vi "Set Position.vi"(8 "error in (no error)":errorcluster, 9 "Datum":T1, 10 "Target Coordinates":T2, 11 "Flex UI (Actor) in":refnum<class "Flex UI (Actor).lvclass">) -> (0 "error out":errorcluster, 3 "Flex UI (Actor) out":refnum<class "Flex UI (Actor).lvclass">)   [LabVIEW 2016, in "Flex UI (Parent Actor).lvlib" / "Flex UI (Actor).lvclass"]
doc: "Wrapper around the set position Flex UI class method."
uses:
  Flex UI (Actor).lvclass
  <vilib>/Utility/miscctls.llb/LVPositionTypeDef.ctl
  <vilib>/East West Architects/Flex UI/Flex UI (Parent)/Enum - Datum.ctl
  <vilib>/East West Architects/Flex UI/Flex UI (Parent)/Flex UI.lvclass
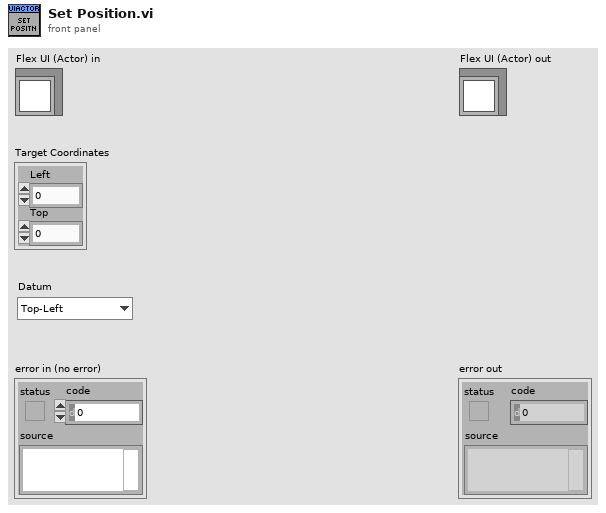
[diagram p1: front panel]
types:
  T1 = typedef "Flex UI.lvclass/Enum - Datum.ctl" = enum16{"Top-Left", "Top-Right", "Bottom-Left", "Bottom-Right", "Center"}
  T2 = typedef "LVPositionTypeDef.ctl" = cluster{"Left":i32, "Top":i32}
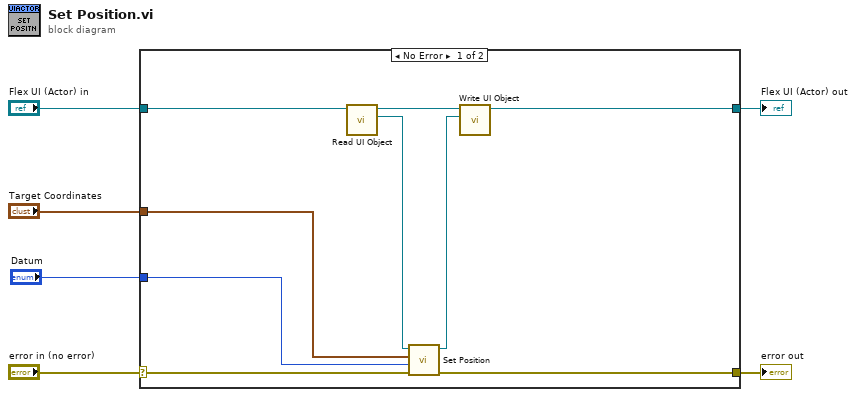
[diagram p0: block diagram]
diagram:
  n1 = case shown="No Error" "error in (no error)" {
    selector: "error in (no error)" -> [w14 w17]
    tunnel: [w13 w17] -> w5
    tunnel: [w10 w16] -> w3
    tunnel: "Flex UI (Actor) in" -> [w15 w16]
    tunnel: "Target Coordinates" -> [w8 _]
    tunnel: "Datum" -> [w7 _]
    frame No Error {
      n2 = call-dynamic "Read UI Object.vi"("Flex UI (Actor) in"=w15) -> ("Flex UI Object"=w11:refnum<class "Flex UI.lvclass">, "Flex UI (Actor) out"=w12:refnum<class "Flex UI (Actor).lvclass">)  [unwired: 8 in, 1 out]
      n3 = call-dynamic "Set Position.vi"("error in"=w14, "Datum"=w7, "Target Coordinates"=w8, "Flex UI in"=w11) -> ("error out"=w13:errorcluster, "Flex UI out"=w9:refnum<class "Flex UI.lvclass">)  [unwired: 6 in]
      n4 = call-dynamic "Write UI Object.vi"("Flex UI in"=w9, "Flex UI (Actor) in"=w12) -> ("Flex UI (Actor) out"=w10:refnum<class "Flex UI (Actor).lvclass">)  [unwired: 8 in, 1 out]
    }
    frame Error {
    }
  }
  "error out" <- w5
  "Flex UI (Actor) out" <- w3
